vi "getCost.vi"(8 "error in (no error)":errorcluster, 11 "HouseBlend in":refnum<class "HouseBlend.lvclass">) -> (0 "error out":errorcluster, 2 "cost":dbl, 3 "HouseBlend out":refnum<class "HouseBlend.lvclass">)   [LabVIEW 2016, in "HouseBlend.lvclass"]
uses:
  HouseBlend.lvclass
  Beverage Class/Beverage.lvclass
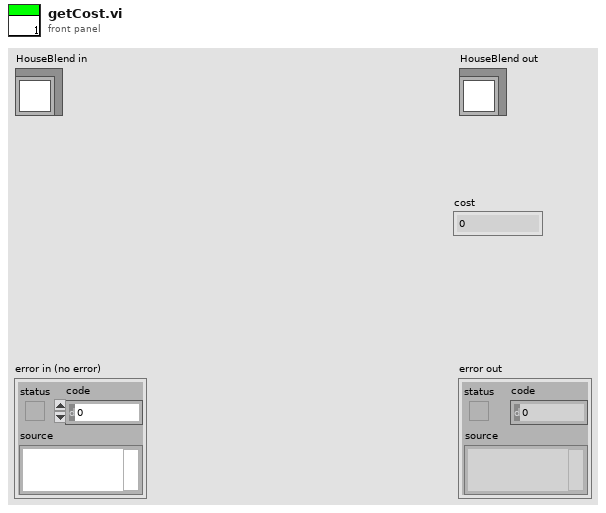
[diagram p1: front panel]
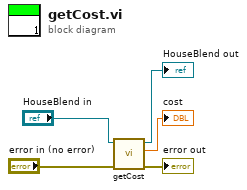
[diagram p0: block diagram]
diagram:
  n1 = call-parent "getCost.vi"("error in (no error)"="error in (no error)", "Beverage in"="HouseBlend in") -> ("error out"=→"error out":errorcluster, "cost"=→"cost":dbl, "Beverage out"=→"HouseBlend out":refnum<class "HouseBlend.lvclass">)  [unwired: 7 in]
